vi "Extract Image Center.vi"(8 "error in (no error)":errorcluster, 9 "y":i32, 10 "x":i32, 11 "Image":T1) -> (0 "error out":errorcluster, 3 "Image out":T1)   [LabVIEW 2012]
uses:
  <vilib>/vision/Image Controls.llb/IMAQ Image.ctl
  <vilib>/vision/NI_Vision_Development_Module.lvlib
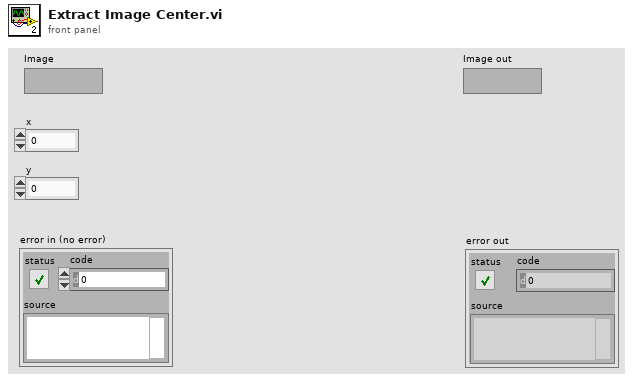
[diagram p1: front panel]
types:
  T1 = typedef "IMAQ Image.ctl" = refnum<image>
  T2 = typedef "Image Type" = u32
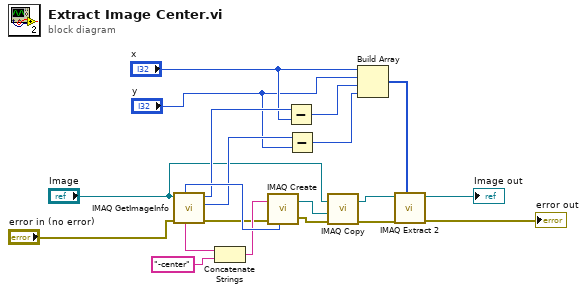
[diagram p0: block diagram]
diagram:
  n1 = call "IMAQ GetImageInfo"("error in (no error)"="error in (no error)", "Image"="Image") -> ("error out"=w16:errorcluster, "Y Resolution"=w10:i32, "X Resolution"=w11:i32, "Image Name"=w19:string, "Image Type"=w20:T2)  [unwired: 2 in, 3 out]
  n2 = Concatenate Strings(w19, "-center" ("string")) -> (w17:string)
  n3 = call "IMAQ Create"("Image Name"=w17, "Image Type"=w20, "error in (no error)"=w16) -> ("New Image"=w5:T1, "error out"=w9:errorcluster)  [unwired: 2 in]
  n4 = Subtract(x=w11, y="x") -> (x-y=w2:i32)
  n5 = Subtract(x=w10, y="y") -> (x-y=w1:i32)
  n6 = call "IMAQ Copy"("error in (no error)"=w9, "Image Dst"=w5, "Image Src"="Image") -> ("error out"=w8:errorcluster, "Image Dst Out"=w7:T1)  [unwired: 3 in]
  n7 = Build Array("x", "y", w2, w1) -> (w12:i32[])
  n8 = call "IMAQ Extract 2"("Optional Rectangle"=w12, "error in (no error)"=w8, "Image Src"=w7) -> ("error out"=→"error out":errorcluster, "Image Dst Out"=→"Image out":T1)  [unwired: 7 in]
